vi "Datacluster remove duplicates_sort.vi"(5 "Remove duplicate":bool, 6 "tolerance":dbl=0.0005 format="%.3e", 7 "ascending":bool, 9 "Sort?":bool, 10 "Datasets to be processed":T1(array[cluster])=[{"String"="sa_cryst,,_2nd.001", "Boolean"=FALSE, "begin"=0, "length"=3962, "y weight"=1.0}, {"String"="sa_cryst,,_2nd.002", "Boolean"=FALSE, "begin"=0, "length"=19075, "y weight"=1.0}, {"String"="sa_cryst,,_2nd.003", "Boolean"=TRUE, "begin"=0, "length"=4476, "y weight"=1.0}], 11 "data cluster":cluster{"all rows":dbl[][]}[](array[cluster])=[{"all rows"=array3962x7[27734 elements]}, {"all rows"=array19075x7[133525 elements]}, {"all rows"=array3233x7[22631 elements]}]) -> (3 "data cluster out":cluster{"all rows":dbl[][]}[](array[cluster]))   [LabVIEW 2020]
panel:
  out "comparative":dbl
  in  "start processing":bool
  in  "target column":u16
  # "(1) Data are sorted ascending or descending order.\n(2) Remove duplicate\n      i) Neighboring two data points are compared, if determined to be a duplicate, the second data point will be removed.\n      ii) Repeat i) unitl no duplicates found."
  # "Caution: All rows will be affected."
  # "(1) Select datasets to be processed"
  # "(2) Sort"
  # "i) Sort ?"
  # "ii) Ascending or descendingwhich order?"
  # "descending"
  # "(3) Remove duplicate? Tolerance?"
  # "(duplicate if \ndata difference <= (max-min) * tolerance"
  # "(4) Start processing"
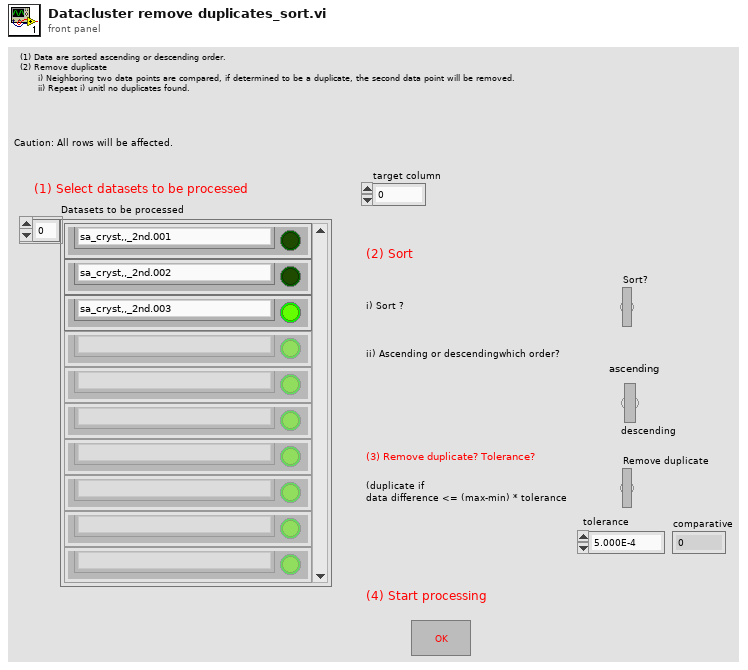
[diagram p1: front panel]
types:
  T1 = cluster{"String":string, "Boolean":bool, "begin":u32, "length":u32, "y weight":dbl}[]
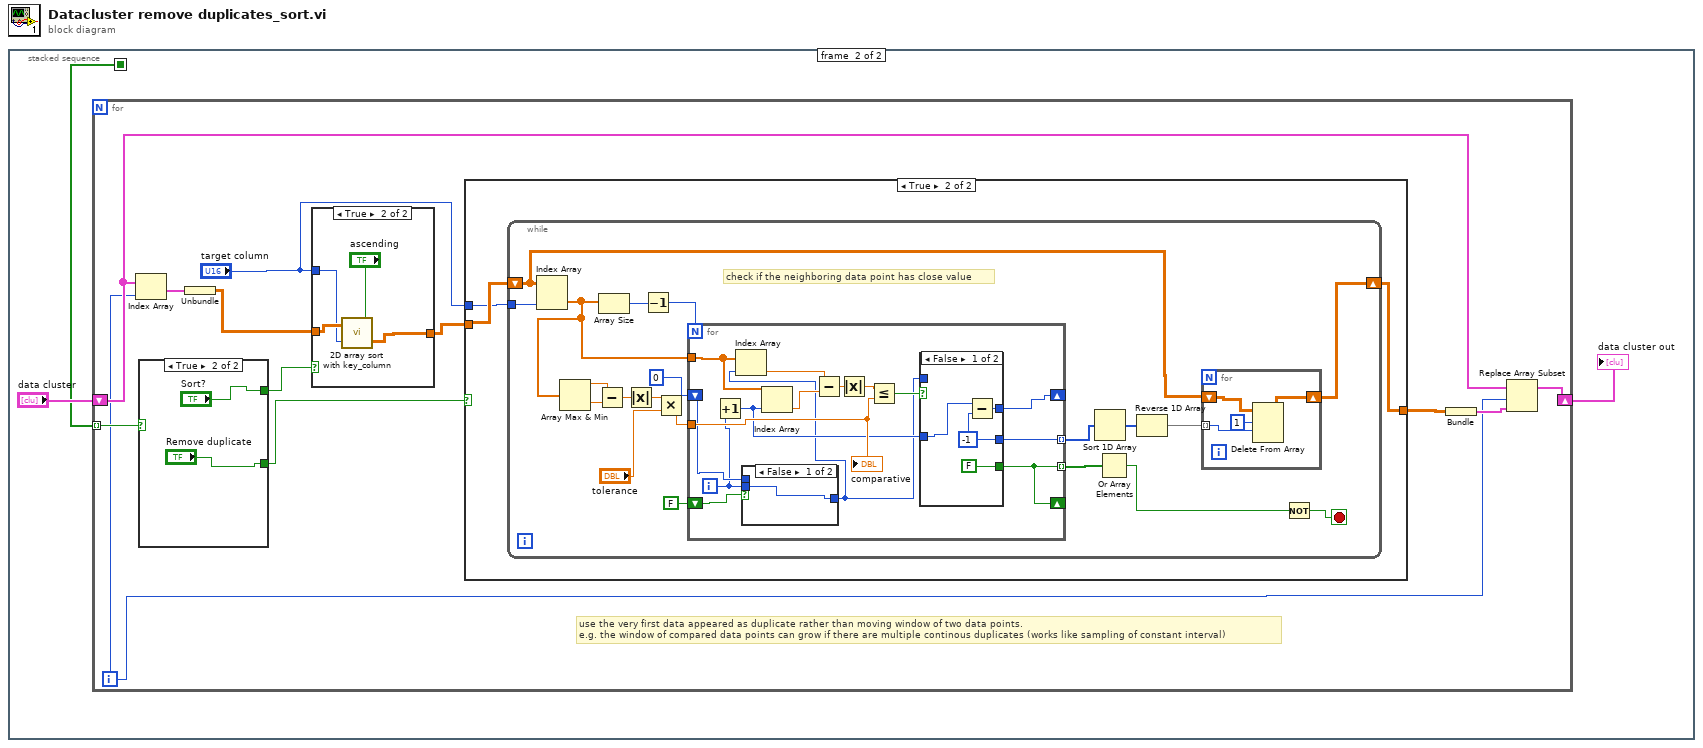
[diagram p0: block diagram]
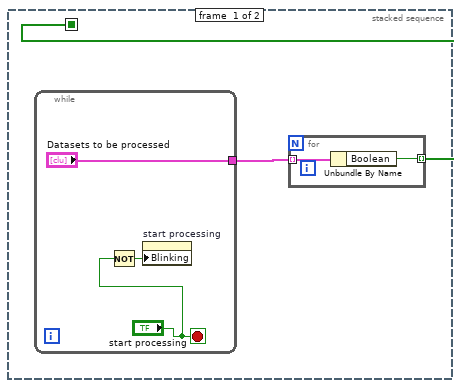
[diagram p2: hidden frame]
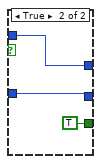
[diagram p5: hidden frame]
diagram:
  n1 = stacked-sequence {
    seq-local: [w1 _] -> [_ w8]
    frame #0 {
      n2 = while {
        tunnel: ["Datasets to be processed"] -> w2
        stop <- "start processing" stop-if-true
        n3 = Not(x="start processing") -> (.not. x?=w6:bool)
        n4 = property on="start processing" class="Bool"("Blinking"=w6) -> ()  [unwired: 2 in, 2 out]
      }
      n5 = for {
        tunnel: w2 -> [w4] mode=indexing
        tunnel: [w3] -> w1 mode=indexing
        n6 = Unbundle By Name(w4) -> ("Boolean"=w3:bool)
      }
    }
    frame #1 {
      n7 = for {
        shift-right: [w15] -> w9
        shift-left: "data cluster" -> [w18]
        tunnel: w8 -> [w14] mode=indexing
        i -> [w12]
        # "use the very first data appeared as duplicate rather than moving window of two data points.\ne.g. the window of compared data points can grow if there are multiple continous duplicates (works like sampling of constant interval)"
        n8 = Index Array(array=w18, index=w12) -> (element=w21:cluster{"all rows":dbl[][]})
        n9 = case shown="True" w14 {
          selector: w14 -> [w75 _]
          tunnel: [w75 "Sort?"] -> w22
          tunnel: [w75 "Remove duplicate"] -> w13
          frame False {
          }
          frame True {
          }
        }
        n10 = Unbundle(w21) -> ("all rows"=w20:dbl[][])
        n11 = case shown="True" w22 {
          tunnel: [w78 w81] -> w19
          tunnel: w20 -> [w78 w82]
          tunnel: "target column" -> [_ w79]
          frame False {
          }
          frame True {
            n12 = call "2D array sort with key_column.vi"("ascending"="ascending", "key column"=w79, "input"=w82) -> ("output"=w81:dbl[][])
          }
        }
        n13 = case shown="True" w13 {
          tunnel: [w23 w24] -> w17
          tunnel: w19 -> [w23 w26]
          tunnel: "target column" -> [_ w25]
          frame False {
          }
          frame True {
            n14 = while {
              tunnel: w25 -> [w40]
              shift-right: [w31] -> w24
              shift-left: w26 -> [w32]
              stop <- w41 stop-if-true
              # "check if the neighboring data point has close value"
              n15 = Index Array(array=w32, index (col)=w40) -> (element=w35:dbl[])  [unwired: 1 in]
              n16 = Array Max & Min(array=w35) -> (max value=w34:dbl, min value=w36:dbl)  [unwired: 2 out]
              n17 = Subtract(x=w34, y=w36) -> (x-y=w37:dbl)
              n18 = Array Size(array=w35) -> (size(s)=w30:i32)
              n19 = Absolute Value(x=w37) -> (abs(x)=w39:dbl)
              n20 = Decrement(x=w30) -> (x-1=w29:i32)
              n21 = Multiply(x=w39, y="tolerance") -> (x*y=w33:dbl)
              n22 = for {
                N: w29 -> [_]
                tunnel: w35 -> [w65]
                tunnel: w33 -> [w61]
                tunnel: [w56] -> w45 mode=indexing
                tunnel: [w57] -> w43 mode=indexing
                shift-right: [w55] -> _
                shift-left: 0 -> [w53]
                shift-right: [w57] -> _
                shift-left: FALSE -> [w54]
                i -> [w51]
                n23 = Increment(x=w51) -> (x+1=w59:i32)
                n24 = case shown="False" w54 {
                  tunnel: [w66 w67] -> w52
                  tunnel: w53 -> [_ w67]
                  tunnel: w51 -> [w66 _]
                  frame False {
                  }
                  frame True {
                  }
                }
                n25 = Index Array(array=w65, index=w52) -> (element=w63:dbl)
                n26 = Index Array(array=w65, index=w59) -> (element=w64:dbl)
                n27 = Subtract(x=w63, y=w64) -> (x-y=w62:dbl)
                n28 = Absolute Value(x=w62) -> (abs(x)=w58:dbl)
                n29 = Less Or Equal?(x=w58, y=w61) -> (x <= y?=w60:bool)
                n30 = case shown="False" w60 {
                  tunnel: w59 -> [w69 w74]
                  tunnel: [w70 w74] -> w56
                  tunnel: [FALSE TRUE] -> w57
                  tunnel: [w68 w72] -> w55
                  tunnel: w52 -> [_ w72]
                  frame False {
                    w70 = -1
                    n31 = Subtract(x=w69, y=w70) -> (x-y=w68:i32)
                  }
                  frame True {
                  }
                }
                "comparative" <- w61
              }
              n32 = Sort 1D Array(array=w45) -> (sorted array=w46:i32[])
              n33 = Or Array Elements(Boolean array=w43) -> (logical OR=w42:bool)
              n34 = Reverse 1D Array(array=w46) -> (reversed array=w44:i32[])
              n35 = for {
                tunnel: w44 -> [w49] mode=indexing
                shift-right: [w47] -> w31
                shift-left: w32 -> [w48]
                n36 = Delete From Array(array=w48, length=1, index (row)=w49) -> (array with subset deleted=w47:dbl[][])  [unwired: 1 in, 1 out]
              }
              n37 = Not(x=w42) -> (.not. x?=w41:bool)
            }
          }
        }
        n38 = Bundle("output"=w17) -> (w16:cluster{"output":dbl[][]})  [unwired: 1 in]
        n39 = Replace Array Subset(array=w18, new element=w16, index=w12) -> (w15:cluster{"all rows":dbl[][]}[])
      }
      "data cluster out" <- w9
    }
  }
